vi "Initialize.vi"() -> (0 "error out":errorcluster, 2 "Wavelength":dbl, 3 "Device Index":u8)   [LabVIEW 2019, in "Topas.lvlib"]
uses:
  Topas.lvlib
  <vilib>/Utility/config.llb/Read Key (String).vi
  Topas-LabVIEW-Driver/TopasDriver.lvlib
  <vilib>/Utility/config.llb/NI_LVConfig.lvlib
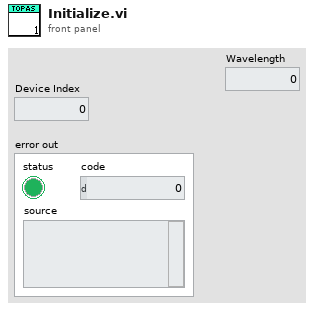
[diagram p1: front panel]
types:
  T1 = typedef "NI_LVConfig.lvlib/Config Data RefNum.ctl" = refnum<k1>
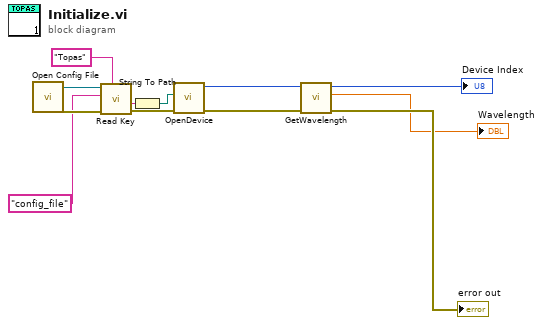
[diagram p0: block diagram]
diagram:
  n1 = call "Open Config File.vi"() -> ("error out"=w10:errorcluster, "Refnum out"=w11:T1)  [unwired: 10 in]
  n2 = call-poly <vilib>:"Read Key.vi"("section"="Topas", "error in (no error)"=w10, "key"="config_file", "refnum"=w11) -> ("error out"=w5:errorcluster, "value"=w9:string)  [unwired: 4 in, 2 out]
  n3 = String To Path(string=w9) -> (path=w8:path)
  n4 = call "OpenDevice.vi"("error in (no error)"=w5, "path"=w8) -> ("error out"=w12:errorcluster, "Device Index"=w3:u8)  [unwired: 8 in]
  n5 = call "GetWavelength.vi"("error in (no error)"=w12, "Device Index"=w3) -> ("error out"=→"error out":errorcluster, "Wavelength"=→"Wavelength":dbl, "Device Index"=→"Device Index":u8)  [unwired: 6 in, 1 out]
